vi "IRDirection_Test.vi"(11 "BrickReferance In":T1) -> (0 "Direction":bool, 3 "BrickReferance out":T1)   [LabVIEW 2012]
uses:
  <vilib>/NXT/Subs/LVHSConnector.ctl
  <vilib>/NXT/LegoClasses/BrickReference/BrickReference.lvclass
  <vilib>/NXT/Block Support/NXT_ButtonSelector.ctl
  <vilib>/NXT/Dual Mode Library/Sensors/readNXTButton.vi
  <vilib>/NXT/Dual Mode Library/Display/drawText.vi
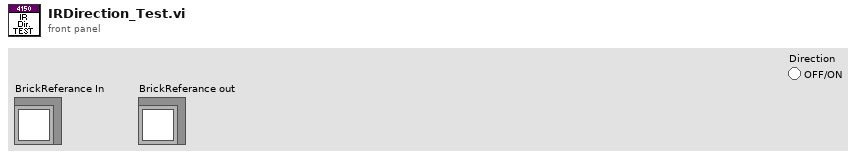
[diagram p1: front panel]
types:
  T1 = typedef "LVHSConnector.ctl" = refnum<class "BrickReference.lvclass">
  T2 = typedef "NXT_ButtonSelector.ctl" = u16
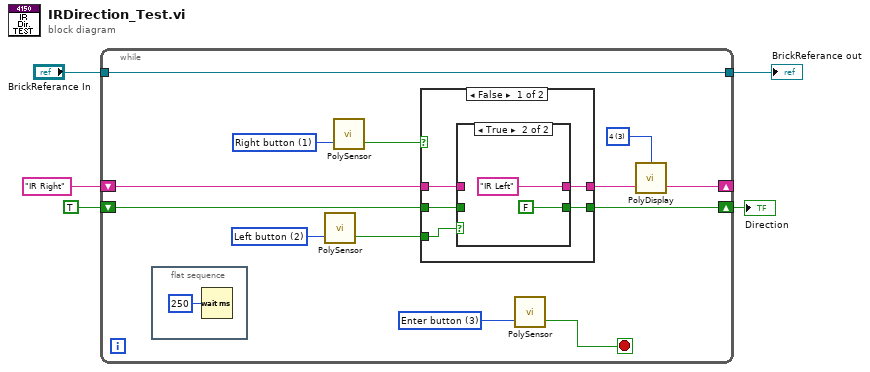
[diagram p0: block diagram]
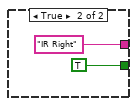
[diagram p3: hidden frame]
diagram:
  n1 = while {
    tunnel: [w17] -> w4
    tunnel: "BrickReferance In" -> [w17]
    shift-right: [w7] -> _
    shift-left: "IR Right" -> [w10]
    shift-right: [w11] -> w1
    shift-left: TRUE -> [w12]
    stop <- w15 stop-if-true
    w6 = i16 3 items=["1", "2", "3", "4", "5", "6", "7", "8"] ("Line")
    w13 = T2 2 items=["Enter button"=3, "Left button"=2, "Right button"=1] ("Button (Enter button)")
    w14 = T2 1 items=["Enter button"=3, "Left button"=2, "Right button"=1] ("Button (Enter button)")
    w16 = T2 3 items=["Enter button"=3, "Left button"=2, "Right button"=1] ("Button (Enter button)")
    n2 = flat-sequence {
      frame #0 {
        n3 = Wait (ms)(milliseconds to wait=u32 250) -> ()  [unwired: 1 out]
      }
    }
    n4 = call-poly <vilib>:"PolySensor.vi"("Button (Enter button)"=w13) -> ("Yes/No"=w8:bool)  [unwired: 2 in, 1 out]
    n5 = call-poly <vilib>:"PolySensor.vi"("Button (Enter button)"=w14) -> ("Yes/No"=w9:bool)  [unwired: 2 in, 1 out]
    n6 = case shown="False" w9 {
      tunnel: [w20 TRUE] -> w11
      tunnel: w12 -> [w21 _]
      tunnel: w10 -> [w19 _]
      tunnel: [w18 "IR Right"] -> w7
      tunnel: w8 -> [w22 _]
      frame False {
        n7 = case shown="True" w22 {
          tunnel: [w23 FALSE] -> w20
          tunnel: w21 -> [w23 _]
          tunnel: [w24 "IR Left"] -> w18
          tunnel: w19 -> [w24 _]
          frame False {
          }
          frame True {
          }
        }
      }
      frame True {
      }
    }
    n8 = call-poly <vilib>:"PolySensor.vi"("Button (Enter button)"=w16) -> ("Yes/No"=w15:bool)  [unwired: 2 in, 1 out]
    n9 = call-poly <vilib>:"PolyDisplay.vi"("Text"=w7, "Line"=w6) -> ()  [unwired: 2 in, 1 out]
  }
  "BrickReferance out" <- w4
  "Direction" <- w1
